vi "Replace BD Constant.vi"(8 "error in (no error)":errorcluster, 11 "Getter Generator In":refnum<class "Getter Generator.lvclass">) -> (0 "error out":errorcluster, 3 "Getter Generator Out":refnum<class "Getter Generator.lvclass">)   [LabVIEW 2020, in "Method Generation.lvlib" / "Getter Generator.lvclass"]
uses:
  Getter Generator.lvclass
  <vilib>/Utility/traverseref.llb/TRef TravTarget.ctl
  Getter Generator.lvclass/Getter Generator.ctl
  <vilib>/Utility/traverseref.llb/VI Scripting - Traverse.lvlib
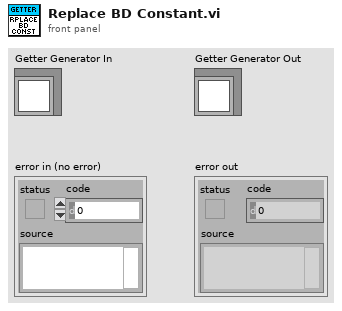
[diagram p1: front panel]
types:
  T1 = typedef "TRef TravTarget.ctl" = enum16{"FP", "BD", "Other"}
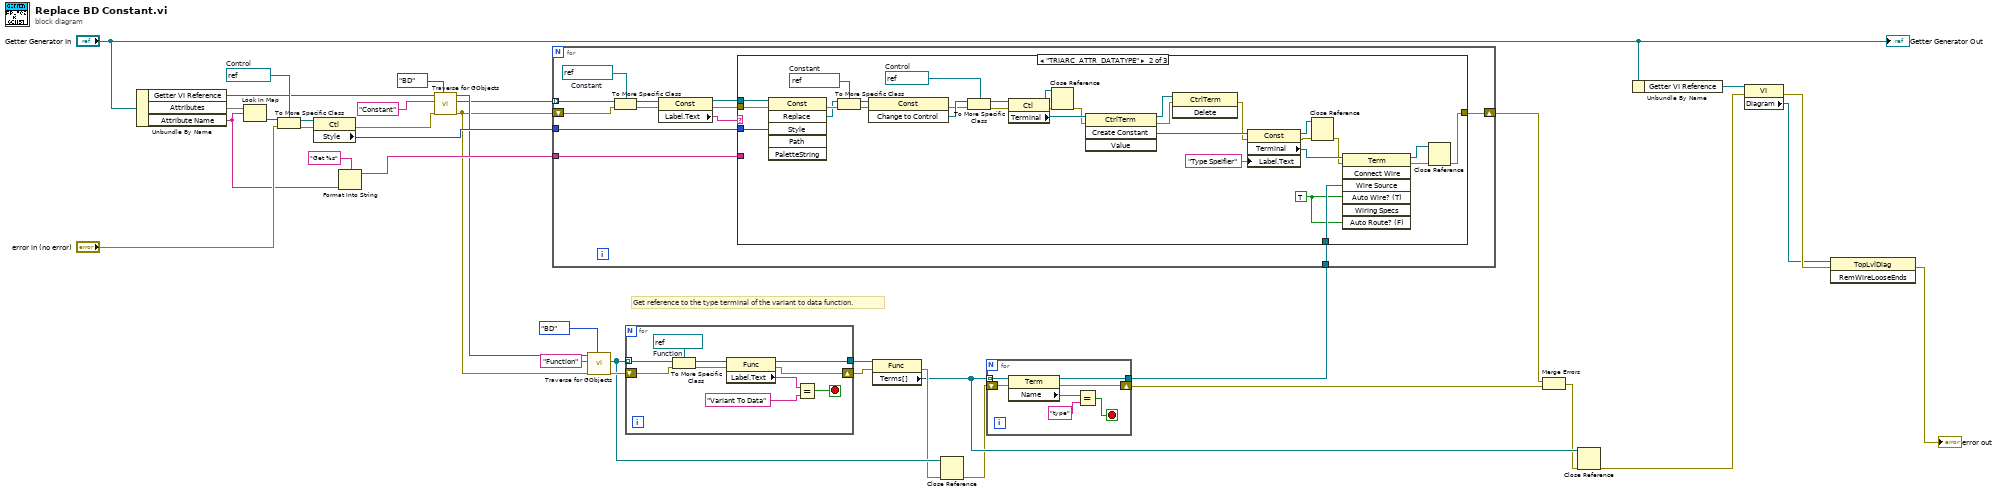
[diagram p0: block diagram]
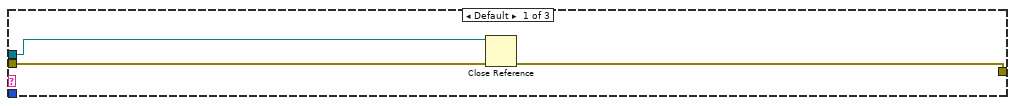
[diagram p2: hidden frame]
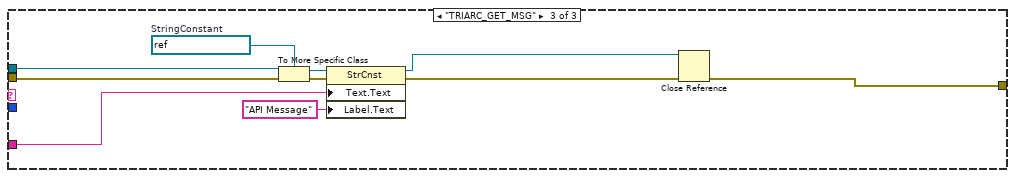
[diagram p3: hidden frame]
diagram:
  w30 = refnum<vi> refnum  # Control
  # "Get reference to the type terminal of the variant to data function."
  n1 = Unbundle By Name("Getter Generator In") -> ("Getter VI Reference"=w22:refnum<vi>, "Attributes"=w33:map{string, refnum<vi>}, "Attribute Name"=w24:string)
  n2 = Look In Map(map=w33, key=w24) -> (value=w32:refnum<vi>)  [unwired: 1 in, 1 out]
  n3 = To More Specific Class(target class=w30, reference=w32, error in="error in (no error)") -> (specific class reference=w31:refnum<vi>, error out=w28:errorcluster)
  n4 = property class="Ctl"(reference=w31, error in=w28) -> (error out=w26:errorcluster, "Style"=w29:u32)  [unwired: 1 out]
  n5 = Format Into String(format string="Get %s", w24) -> (resulting string=w23:string)  [unwired: 2 in, 1 out]
  n6 = call <vilib>:"Traverse for GObjects.vi"("Traverse Target"=TRef_TravTarget."BD", "error in (no error)"=w26, "Class Name"="Constant", "VI Refnum"=w22) -> ("error out"=w10:errorcluster, "References"=w19:refnum<vi>[])  [unwired: 4 in, 2 out]
  n7 = call <vilib>:"Traverse for GObjects.vi"("Traverse Target"=TRef_TravTarget."BD", "error in (no error)"=w10, "Class Name"="Function", "VI Refnum"=w22) -> ("error out"=w16:errorcluster, "References"=w15:refnum<vi>[])  [unwired: 4 in, 2 out]
  n8 = for {
    tunnel: w15 -> [w45] mode=indexing
    tunnel: [w42] -> w18
    shift-right: [w36] -> w14
    shift-left: w16 -> [w38]
    stop <- w39 stop-if-true
    w44 = refnum<vi> refnum  # Function
    n9 = To More Specific Class(target class=w44, reference=w45, error in=w38) -> (specific class reference=w43:refnum<vi>, error out=w37:errorcluster)
    n10 = property class="Func"(reference=w43, error in=w37) -> (reference out=w42:refnum<vi>, error out=w36:errorcluster, "Label.Text"=w41:string)
    n11 = Equal?(x=w41, y="Variant To Data") -> (x = y?=w39:bool)
  }
  n12 = property class="Func"(reference=w18, error in=w14) -> (error out=w13:errorcluster, "Terms[]"=w12:refnum<vi>[])  [unwired: 1 out]
  n13 = Close Reference(reference=w15, error in (no error)=w13) -> (error out=w9:errorcluster)
  n14 = for {
    tunnel: w12 -> [w52] mode=indexing
    tunnel: [w49] -> w17
    shift-right: [w46] -> w8
    shift-left: w9 -> [w47]
    stop <- w48 stop-if-true
    n15 = property class="Term"(reference=w52, error in=w47) -> (reference out=w49:refnum<vi>, error out=w46:errorcluster, "Name"=w51:string)
    n16 = Equal?(x=w51, y="type") -> (x = y?=w48:bool)
  }
  n17 = for {
    tunnel: w19 -> [w64] mode=indexing
    tunnel: w29 -> [w62]
    shift-right: [w61] -> w6
    shift-left: w10 -> [w63]
    tunnel: w23 -> [w54]
    tunnel: w17 -> [w53]
    w60 = refnum<vi> refnum  # Constant
    n18 = To More Specific Class(target class=w60, reference=w64, error in=w63) -> (specific class reference=w57:refnum<vi>, error out=w59:errorcluster)
    n19 = property class="Const"(reference=w57, error in=w59) -> (reference out=w56:refnum<vi>, error out=w58:errorcluster, "Label.Text"=w55:string)
    n20 = case shown="\"TRIARC_ATTR_DATATYPE\"" w55 {
      tunnel: w62 -> [_ w98 _]
      tunnel: [w66 w72 w101] -> w61
      tunnel: w58 -> [w67 w97 w107]
      tunnel: w56 -> [w65 w89 w108]
      tunnel: w54 -> [_ _ w103]
      tunnel: w53 -> [_ w80 _]
      frame Default {
        n21 = Close Reference(reference=w65, error in (no error)=w67) -> (error out=w66:errorcluster)
      }
      frame "TRIARC_ATTR_DATATYPE" {
        w79 = TRUE ("Auto Wire? (T)")
        w84 = refnum<vi> refnum  # Constant
        w96 = refnum<vi> refnum  # Control
        n22 = invoke class="Const" method="Replace"(reference=w89, error in=w97, "Style"=w98) -> (error out=w93:errorcluster, "Replace"=w86:refnum<vi>)  [unwired: 3 in, 4 out]
        n23 = To More Specific Class(target class=w84, reference=w86, error in=w93) -> (specific class reference=w85:refnum<vi>, error out=w87:errorcluster)
        n24 = invoke class="Const" method="Change to Control"(reference=w85, error in=w87) -> (error out=w75:errorcluster, "Change to Control"=w83:refnum<vi>)  [unwired: 1 in, 1 out]
        n25 = To More Specific Class(target class=w96, reference=w83, error in=w75) -> (specific class reference=w95:refnum<vi>, error out=w92:errorcluster)
        n26 = property class="Ctl"(reference=w95, error in=w92) -> (reference out=w73:refnum<vi>, error out=w88:errorcluster, "Terminal"=w94:refnum<vi>)
        n27 = Close Reference(reference=w73, error in (no error)=w88) -> (error out=w74:errorcluster)
        n28 = invoke class="CtrlTerm" method="Create Constant"(reference=w94, error in=w74) -> (reference out=w91:refnum<vi>, error out=w90:errorcluster, "Create Constant"=w82:refnum<vi>)  [unwired: 2 in, 1 out]
        n29 = invoke class="CtrlTerm" method="Delete"(reference=w91, error in=w90) -> (error out=w78:errorcluster)  [unwired: 1 in, 2 out]
        n30 = property class="Const"(reference=w82, error in=w78, "Label.Text"="Type Speifier") -> (reference out=w69:refnum<vi>, error out=w77:errorcluster, "Terminal"=w81:refnum<vi>)
        n31 = Close Reference(reference=w69, error in (no error)=w77) -> (error out=w70:errorcluster)
        n32 = invoke class="Term" method="Connect Wire"(reference=w81, error in=w70, "Wire Source"=w80, "Auto Wire? (T)"=w79, "Auto Route? (F)"=w79) -> (reference out=w71:refnum<vi>, error out=w76:errorcluster)  [unwired: 2 in, 5 out]
        n33 = Close Reference(reference=w71, error in (no error)=w76) -> (error out=w72:errorcluster)
      }
      frame "TRIARC_GET_MSG" {
        w106 = refnum<vi> refnum  # StringConstant
        n34 = To More Specific Class(target class=w106, reference=w108, error in=w107) -> (specific class reference=w105:refnum<vi>, error out=w104:errorcluster)
        n35 = property class="StrCnst"(reference=w105, error in=w104, "Text.Text"=w103, "Label.Text"="API Message") -> (reference out=w100:refnum<vi>, error out=w102:errorcluster)
        n36 = Close Reference(reference=w100, error in (no error)=w102) -> (error out=w101:errorcluster)
      }
    }
  }
  n37 = Merge Errors(w6, w8) -> (w7:errorcluster)
  n38 = Close Reference(reference=w12, error in (no error)=w7) -> (error out=w11:errorcluster)
  n39 = Unbundle By Name("Getter Generator In") -> ("Getter VI Reference"=w3:refnum<vi>)
  n40 = property class="VI"(reference=w3, error in=w11) -> (error out=w4:errorcluster, "Diagram"=w1:refnum<vi>)  [unwired: 1 out]
  n41 = invoke class="TopLvlDiag" method="RemWireLooseEnds"(reference=w1, error in=w4) -> (error out=→"error out":errorcluster)  [unwired: 1 in, 2 out]
  "Getter Generator Out" <- "Getter Generator In"
